vi "LinearQuadraticRegulator_New.vi"(5 "States":i32, 6 "dt_Seconds":dbl=0.02, 7 "Inputs":i32, 8 "R":T1, 9 "Q":T1, 10 "B":T1, 11 "A":T1) -> (0 "Error":errorcluster, 3 "LinearQuadraticRegulator":T2)   [LabVIEW 2019, in "Trajectory_Library.lvlib"]
doc: "Contains the controller coefficients and logic for a linear-quadratic regulator (LQR). LQRs use the control law u = K(r - x).\n \nFor more on the underlying math, read https://file.tavsys.net/control/controls-engineering-in-frc.pdf.\n\nConstructs a controller with the given coefficients and plant.\n\nInputs:\n - A -- Continuous system matrix of the plant being controlled.\n - B -- Continuous input matrix of the plant being controlled.\n - Q -- The state cost matrix.\n - R -- The input cost matrix.\n - dtSeconds -- Discretization timestep.\n\nOutputs:\n - LinearQuadraticRegulator -- controller data cluster\n - Error -- if TRUE, and error occured"
uses:
  Trajectory_Library.lvlib
  <vilib>/Analysis/Matrix/Datatypes/RealMatrix.ctl
  <vilib>/Analysis/Matrix/NI_Matrix.lvlib
  TypeDef/LINEAR_QUADRATIC_REGULATOR.ctl
  <vilib>/Analysis/NI_AALPro.lvlib
  <vilib>/Analysis/NI_AALBase.lvlib
  <vilib>/Analysis/baseanly.llb/Real A x B.vi
  <vilib>/Analysis/7linalg.llb/Solve Linear Equations (multiple right hand).vi
  <vilib>/Analysis/Matrix/Numeric/Add/Add - RM,RM.vi
  <vilib>/Analysis/7linalg.llb/Real Transpose Matrix.vi
panel:
  # "<States,States>"
  # "<States,Inputs>"
  # "<States,States>"
  # "<Inputs,Inputs>"
  # "Ref State <States,1>"
  # "Comp and capped \noutput <Inputs,1>"
  # "Controller gain\n<Inputs,States>"
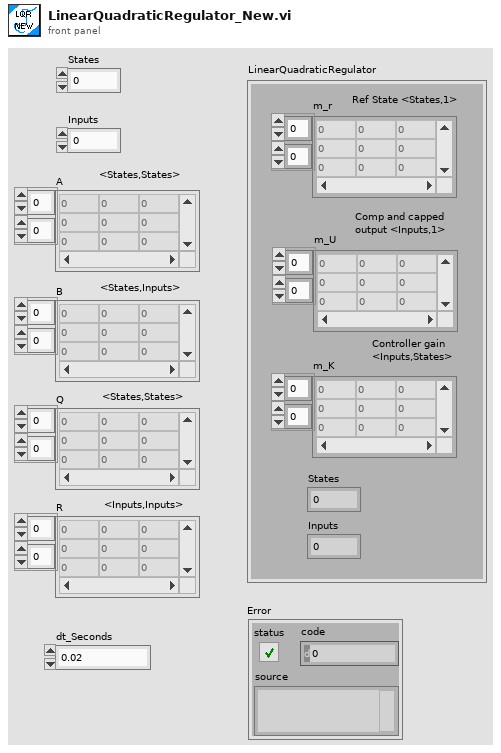
[diagram p1: front panel]
types:
  T1 = typedef "NI_Matrix.lvlib/RealMatrix.ctl" = dbl[][]
  T2 = typedef "Trajectory_Library.lvlib/LINEAR_QUADRATIC_REGULATOR.ctl" = cluster{"m_r":T1, "m_U":T1, "m_K":T1, "States":i32, "Inputs":i32}
  T3 = typedef "WPILib_Math.lvlib/LINEAR_QUADRATIC_REGULATOR.ctl" = cluster{"m_r":T1, "m_U":T1, "m_K":T1, "States":i32, "Inputs":i32}
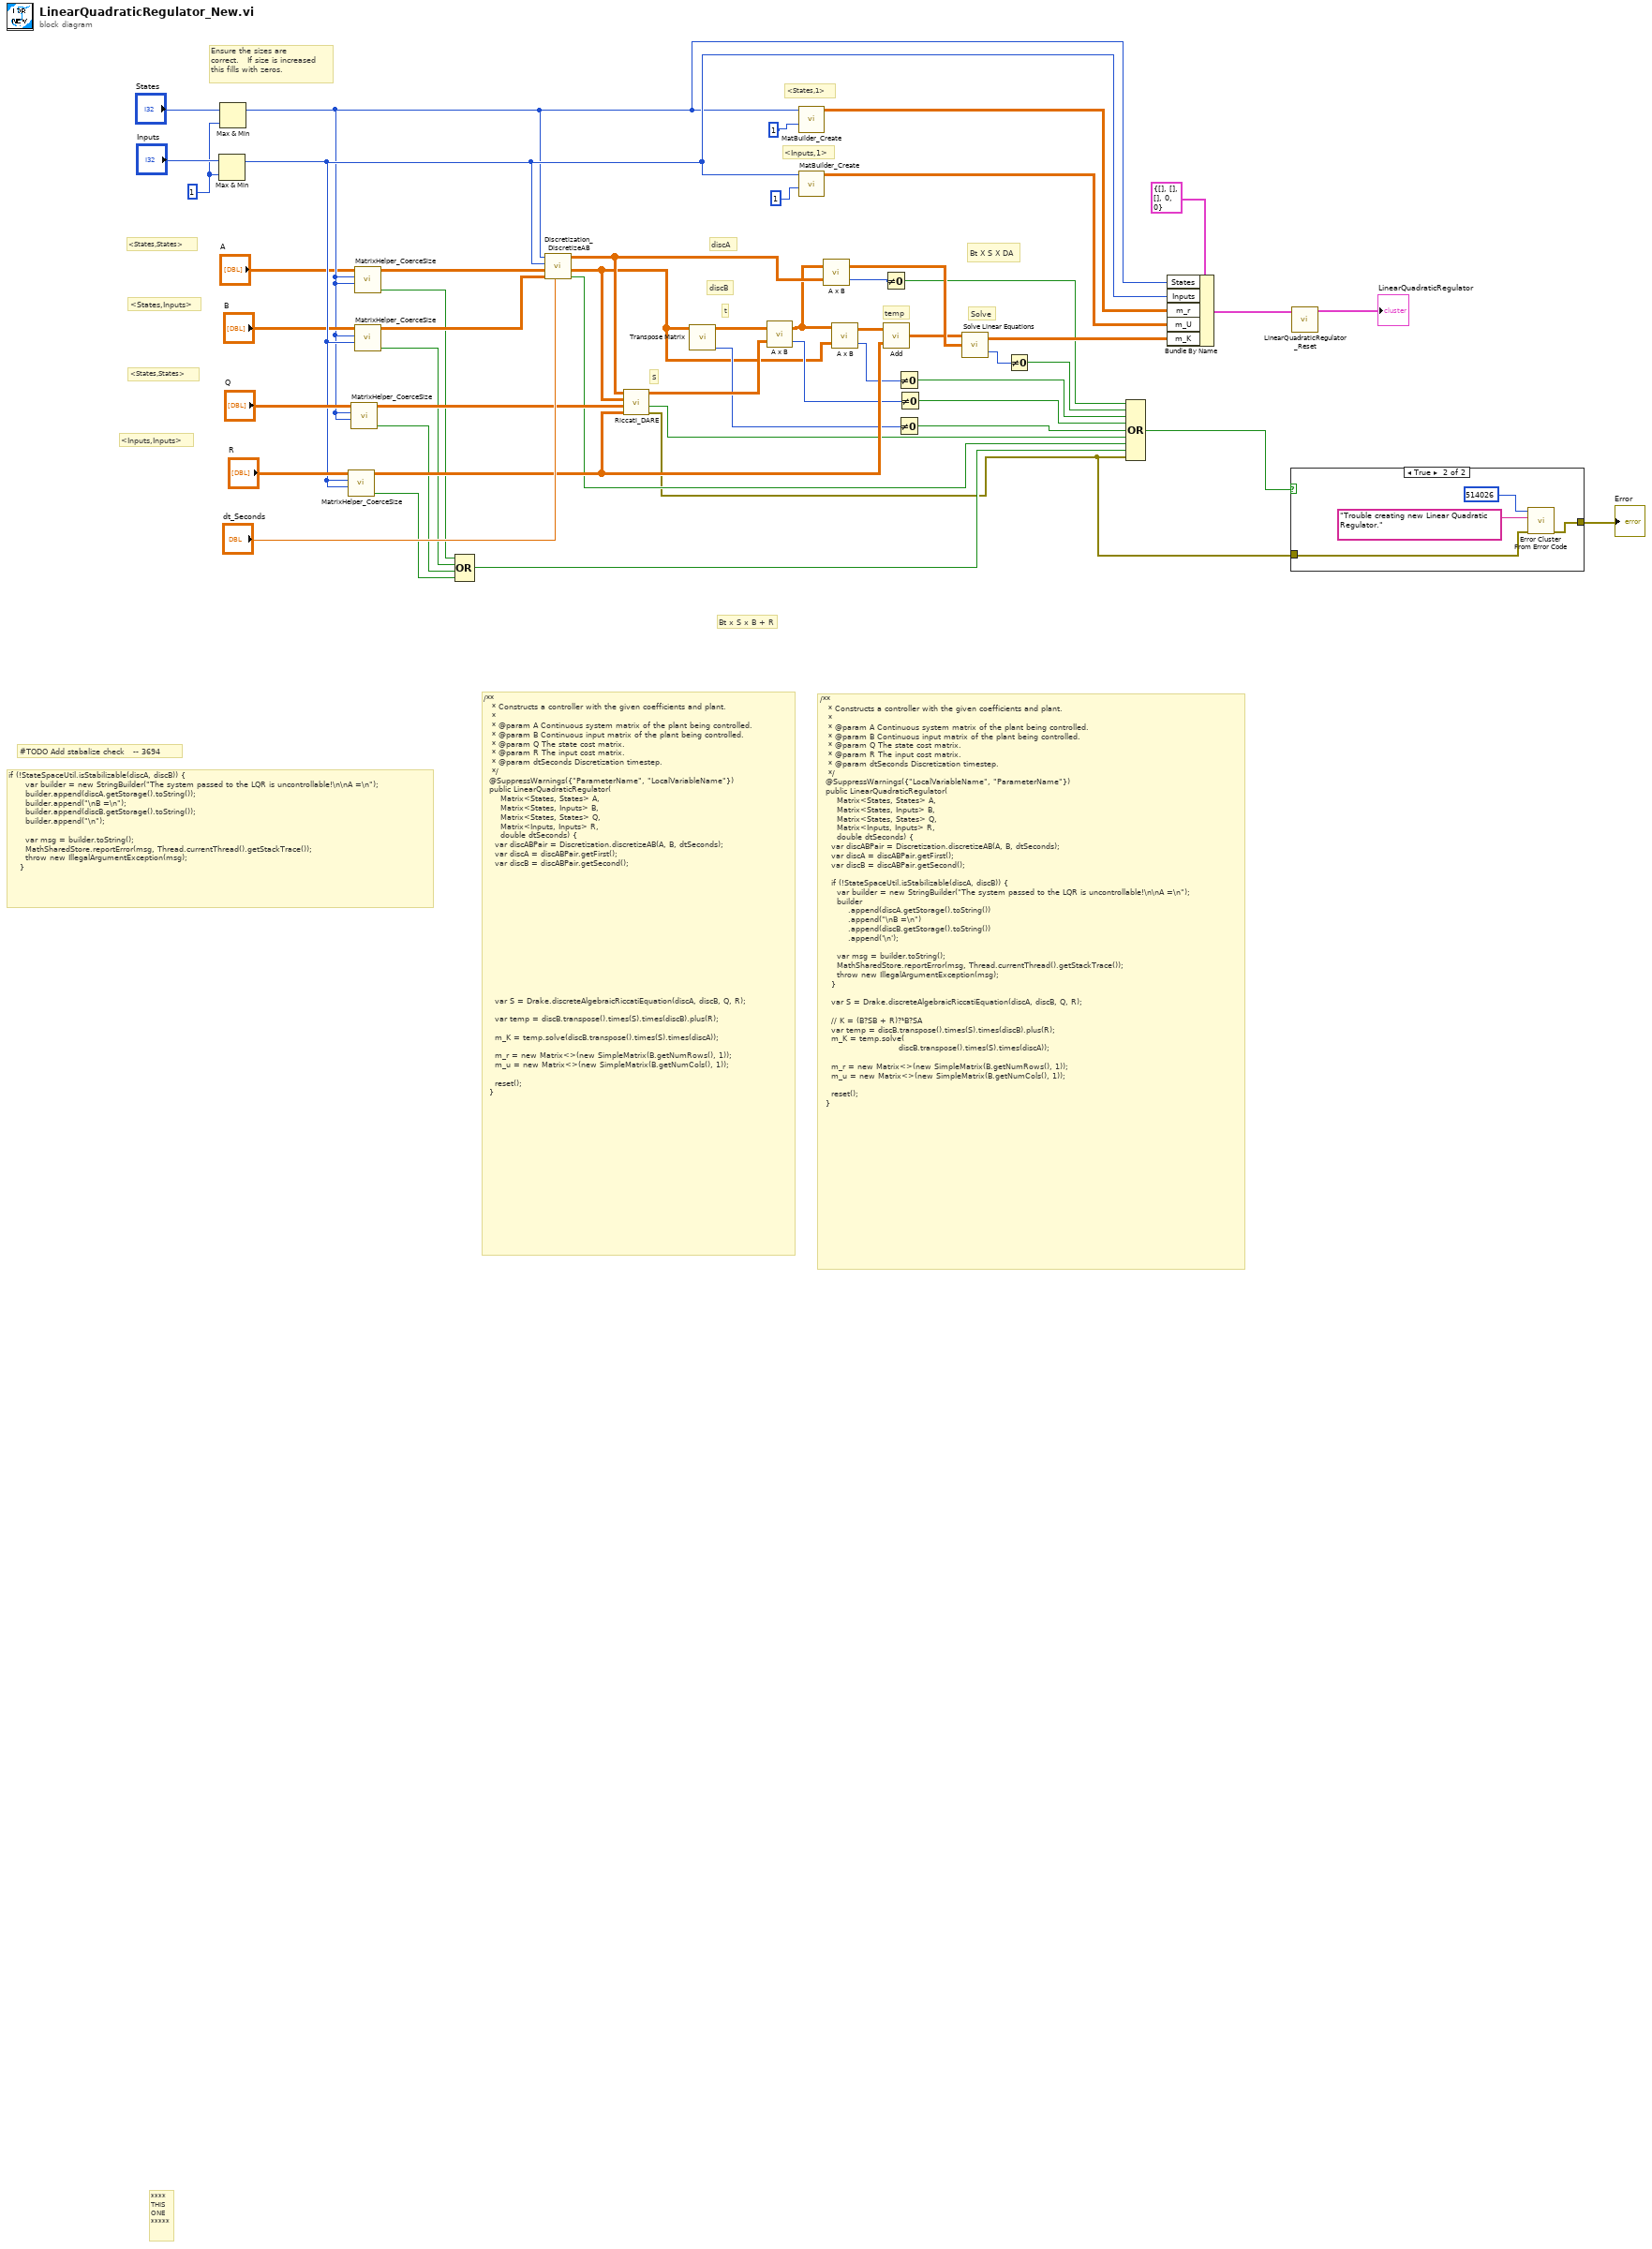
[diagram p0: block diagram]
diagram:
  w47 = 1 ("y")
  # "/**\n   * Constructs a controller with the given coefficients and plant.\n   *\n   * @param A Continuous system matrix of the plant being controlled.\n   * @param B Continuous input matrix of the plant being controlled.\n   * @param Q The state cost matrix.\n   * @param R The input cost matrix.\n   * @param dtSeconds Discretization timestep.\n   */\n  @SuppressWarnings({\"LocalVariableName\", \"ParameterName\"})\n  public LinearQuadraticRegulator(\n      Matrix<States, States> A,\n      Matrix<States, Inputs> B,\n      Matrix<States, States> Q,\n      Matrix<Inputs, Inputs> R,\n      double dtSeconds) {\n    var discABPair = Discretization.discretizeAB(A, B, dtSeconds);\n    var discA = discABPair.getFirst();\n    var discB = discABPair.getSecond();\n\n    if (!StateSpaceUtil.isStabilizable(discA, discB)) {\n      var builder = new StringBuilder(\"The system passed to the LQR is uncontrollable!\\n\\nA =\\n\");\n      builder\n          .append(discA.getStorage().toString())\n          .append(\"\\nB =\\n\")\n          .append(discB.getStorage().toString())\n          .append('\\n');\n\n      var msg = builder.toString();\n      MathSharedStore.reportError(msg, Thread.currentThread().getStackTrace());\n      throw new IllegalArgumentException(msg);\n    }\n\n    var S = Drake.discreteAlgebraicRiccatiEquation(discA, discB, Q, R);\n\n    // K = (B?SB + R)?¹B?SA\n    var temp = discB.transpose().times(S).times(discB).plus(R);\n    m_K = temp.solve(\n                            discB.transpose().times(S).times(discA));\n\n    m_r = new Matrix<>(new SimpleMatrix(B.getNumRows(), 1));\n    m_u = new Matrix<>(new SimpleMatrix(B.getNumCols(), 1));\n\n    reset();\n  }"
  # "#TODO Add stabalize check   -- 3694"
  # "if (!StateSpaceUtil.isStabilizable(discA, discB)) {\n      var builder = new StringBuilder(\"The system passed to the LQR is uncontrollable!\\n\\nA =\\n\");\n      builder.append(discA.getStorage().toString());\n      builder.append(\"\\nB =\\n\");\n      builder.append(discB.getStorage().toString());\n      builder.append(\"\\n\");\n\n      var msg = builder.toString();\n      MathSharedStore.reportError(msg, Thread.currentThread().getStackTrace());\n      throw new IllegalArgumentException(msg);\n    }"
  # "Bt X S X DA"
  # "Bt x S x B + R"
  # "S"
  # "Solve"
  # "t"
  # "temp"
  # "<Inputs,1>"
  # "<States,1>"
  # "discB"
  # "discA"
  # "<Inputs,Inputs>"
  # "<States,States>"
  # "<States,Inputs>"
  # "<States,States>"
  # "Ensure the sizes are\ncorrect.   If size is increased \nthis fills with zeros."
  # "/**\n   * Constructs a controller with the given coefficients and plant.\n   *\n   * @param A Continuous system matrix of the plant being controlled.\n   * @param B Continuous input matrix of the plant being controlled.\n   * @param Q The state cost matrix.\n   * @param R The input cost matrix.\n   * @param dtSeconds Discretization timestep.\n   */\n  @SuppressWarnings({\"ParameterName\", \"LocalVariableName\"})\n  public LinearQuadraticRegulator(\n      Matrix<States, States> A,\n      Matrix<States, Inputs> B,\n      Matrix<States, States> Q,\n      Matrix<Inputs, Inputs> R,\n      double dtSeconds) {\n    var discABPair = Discretization.discretizeAB(A, B, dtSeconds);\n    var discA = discABPair.getFirst();\n    var discB = discABPair.getSecond();\n\n\n\n\n\n\n\n\n\n\n\n\n\n\n    var S = Drake.discreteAlgebraicRiccatiEquation(discA, discB, Q, R);\n\n    var temp = discB.transpose().times(S).times(discB).plus(R);\n\n    m_K = temp.solve(discB.transpose().times(S).times(discA));\n\n    m_r = new Matrix<>(new SimpleMatrix(B.getNumRows(), 1));\n    m_u = new Matrix<>(new SimpleMatrix(B.getNumCols(), 1));\n\n    reset();\n  }"
  # "****\nTHIS\nONE\n*****"
  n1 = Max & Min(x="Inputs", y=w47) -> (max(x,y)=w38:i32)  [unwired: 1 out]
  n2 = Max & Min(x="States", y=w47) -> (max(x,y)=w35:i32)  [unwired: 1 out]
  n3 = call "MatrixHelper_CoerceSize.vi"("Columns"=w38, "Rows"=w38, "input matrix"="R") -> ("Coerced"=w42:bool, "output matrix"=w43:T1)  [unwired: 7 in]
  n4 = call "MatrixHelper_CoerceSize.vi"("Columns"=w35, "Rows"=w35, "input matrix"="Q") -> ("Coerced"=w39:bool, "output matrix"=w40:T1)  [unwired: 7 in]
  n5 = call "MatrixHelper_CoerceSize.vi"("Columns"=w35, "Rows"=w35, "input matrix"="A") -> ("Coerced"=w31:bool, "output matrix"=w33:T1)  [unwired: 7 in]
  n6 = call "MatrixHelper_CoerceSize.vi"("Columns"=w38, "Rows"=w35, "input matrix"="B") -> ("Coerced"=w32:bool, "output matrix"=w36:T1)  [unwired: 7 in]
  n7 = Compound Arithmetic op=OR(w31, w32, w39, w42) -> (w4:bool)
  n8 = call "Discretization_DiscretizeAB.vi"("dT_Seconds"="dt_Seconds", "ContB"=w36, "ContA"=w33, "Inputs"=w38, "States"=w35) -> ("Error"=w11:bool, "DiscB"=w5:T1, "DiscA"=w26:T1)  [unwired: 4 in]
  n9 = call "Riccati_DARE.vi"("R"=w43, "Q"=w40, "B"=w5, "A"=w26) -> ("error out"=w2:errorcluster, "Error"=w10:bool, "Answer"=w25:T1)  [unwired: 4 in, 1 out]
  n10 = call-poly <vilib>:"Transpose Matrix.vi"("Input Matrix"=w5) -> ("error"=w13:i32, "Matrix Transpose"=w29:T1)  [unwired: 9 in]
  n11 = call-poly <vilib>:"A x B.vi"("B"=w25, "A"=w29) -> ("error"=w15:i32, "A x B"=w24:T1)
  n12 = call "MatBuilder_Create.vi"("Columns"=1 ("number of columns"), "Rows"=w35) -> ("output matrix"=w8:T1)  [unwired: 9 in]
  n13 = call "MatBuilder_Create.vi"("Columns"=1 ("number of columns"), "Rows"=w38) -> ("output matrix"=w7:T1)  [unwired: 9 in]
  n14 = call-poly <vilib>:"A x B.vi"("B"=w26, "A"=w24) -> ("error"=w21:i32, "A x B"=w28:T1)
  n15 = call-poly <vilib>:"A x B.vi"("B"=w5, "A"=w24) -> ("error"=w20:i32, "A x B"=w23:T1)
  n16 = Not Equal To 0?(x=w21) -> (x != 0?=w18:bool)
  n17 = call-poly <vilib>:"Add.vi"("Real Matrix B"=w43, "Real Matrix A"=w23) -> ("A + B"=w22:T1)
  n18 = Not Equal To 0?(x=w20) -> (x != 0?=w16:bool)
  n19 = Not Equal To 0?(x=w13) -> (x != 0?=w12:bool)
  n20 = Not Equal To 0?(x=w15) -> (x != 0?=w14:bool)
  n21 = call-poly <vilib>:"Solve Linear Equations.vi"("Known Matrix"=w28, "Input Matrix"=w22) -> ("error"=w19:i32, "Solution Matrix"=w27:T1)  [unwired: 1 in]
  n22 = Not Equal To 0?(x=w19) -> (x != 0?=w17:bool)
  n23 = Compound Arithmetic op=OR(w18, w17, w16, w14, w12, w10, w11, w4, w2) -> (w3:bool)
  n24 = Bundle By Name(cluster=T2 {"m_r"=[], "m_U"=[], "m_K"=[], "States"=0, "Inputs"=0} ("LINEARQUADRATICREGULATOR"), "States"=w35, "Inputs"=w38, "m_r"=w8, "m_U"=w7, "m_K"=w27) -> (w46:T2)
  n25 = case shown="True" w3 {
    tunnel: w2 -> [w51 w54]
    tunnel: [w51 w55] -> w1
    frame False {
    }
    frame True {
      n26 = call <vilib>:"Error Cluster From Error Code.vi"("error in (no error)"=w54, "error message (\"\")"="Trouble creating new Linear Quadratic Regulator." ("error message (\"\")"), "error code (0)"=514026) -> ("error out"=w55:errorcluster)  [unwired: 6 in]
    }
  }
  "Error" <- w1
  n27 = call "LinearQuadraticRegulator_Reset.vi"("in LinearQuadraticRegulator"=w46) -> ("out LinearQuadraticRegulator"=→"LinearQuadraticRegulator":T3)  [unwired: 10 in]
